vi "Write Singleton.vi"(8 "error in (no error)":errorcluster, 11 "Class in":refnum<class>) -> (0 "error out":errorcluster)   [LabVIEW 2020, in "Singleton.lvlib"]
uses:
  Singleton.lvlib
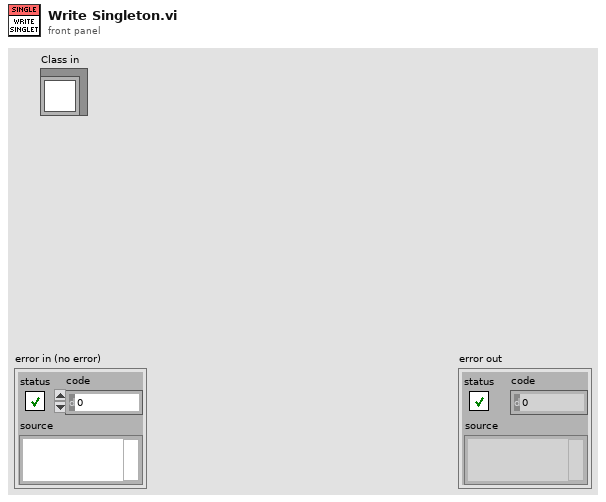
[diagram p1: front panel]
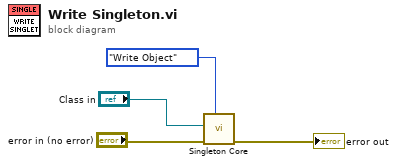
[diagram p0: block diagram]
diagram:
  n1 = call "Singleton Core.vi"("Action"=enum16{"Init", "Write Object", "Read Object"}."Write Object", "error in (no error)"="error in (no error)", "Class in"="Class in") -> ("error out"=→"error out":errorcluster)  [unwired: 7 in, 1 out]
